vi "Sr530 ReadCh.vi"(0 "VISA Rsrc":refnum<visa-resource-name>="SR530", 1 "Autoscale":bool=TRUE, 5 "Channel":T1 items=["Channel 1", "X Output", "Channel 2", "Y Output", "X1", "X2", "X3", "X4", "X5", "X6", "Ch1 and Ch2", "X and Y", "X,Y,Ch1,Ch2"], 7 "Délais":u32, 9 "Check Status":bool, 11 "error in (no error)":errorcluster, 12 "Ask Correction":bool) -> (2 "Outputs":dbl[](array[numeric]), 3 "Warning":bool, 4 "Ressource VISA Out":refnum<visa-resource-name>="GPIB0::8::INSTR", 6 "Output":dbl format="%.4e", 8 "Output 2":dbl format="%.4e", 10 "Status Byte":bool[](array[boolean]), 14 "Ask Correction Out":bool, 15 "error out":errorcluster)   [LabVIEW 2019]
uses:
  <userlib>/SR530/Inputs.ctl
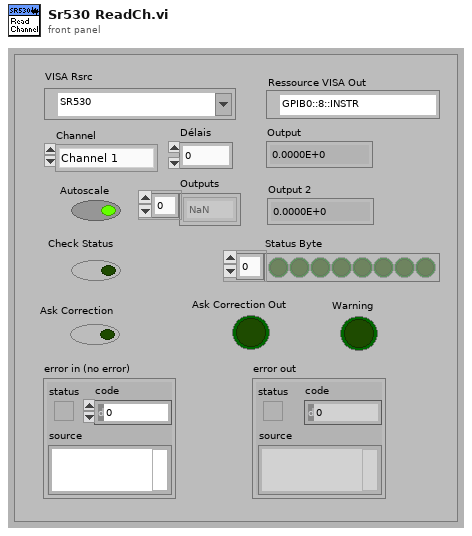
[diagram p1: front panel]
types:
  T1 = typedef "Inputs.ctl" = u16
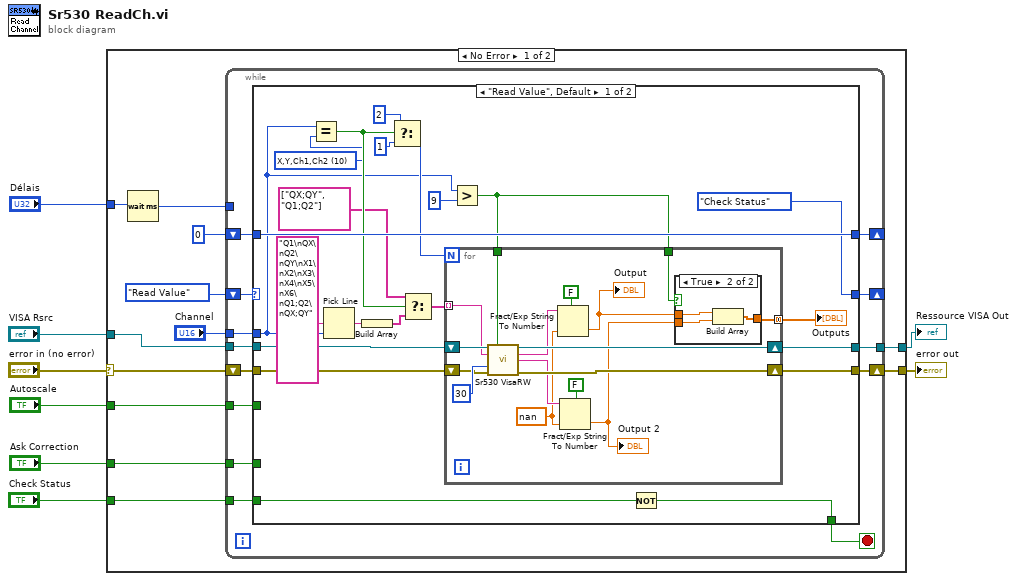
[diagram p0: block diagram]
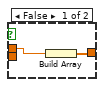
[diagram p2: hidden frame]
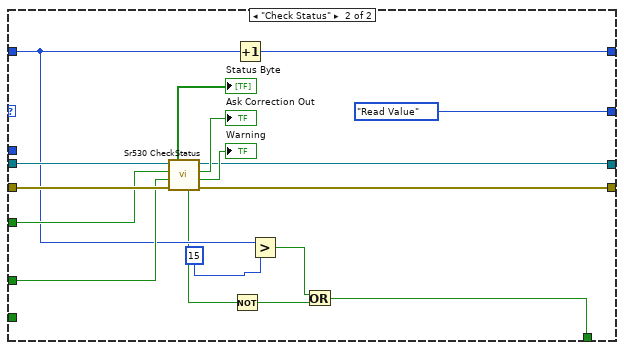
[diagram p3: hidden frame]
diagram:
  n1 = case shown="No Error" "error in (no error)" {
    selector: "error in (no error)" -> [w13 w95]
    tunnel: [w19 w95] -> w7
    tunnel: "Autoscale" -> [w18 _]
    tunnel: "Check Status" -> [w15 _]
    tunnel: "VISA Rsrc" -> [w14 w94]
    tunnel: "Ask Correction" -> [w12 _]
    tunnel: [w11 w94] -> w2
    tunnel: "Délais" -> [w10 _]
    frame No Error {
      n2 = Wait (ms)(milliseconds to wait=w10) -> (millisecond timer value=w9:u32)
      n3 = while {
        shift-right: [w29] -> _
        shift-left: enum16{"Read Value", "Check Status"}."Read Value" -> [w33]
        shift-right: [w31] -> w19
        shift-left: w13 -> [w32]
        tunnel: w18 -> [w28]
        tunnel: "Channel" -> [w27]
        shift-right: [w25] -> _
        shift-left: 0 ("timeout ms (488.2 global)") -> [w26]
        tunnel: w15 -> [w24]
        tunnel: w14 -> [w23]
        tunnel: w12 -> [w22]
        tunnel: [w21] -> w11
        tunnel: w9 -> [_]
        stop <- w30 stop-if-true
        n4 = case shown="\"Read Value\", Default" w33 {
          tunnel: w32 -> [w48 w93]
          tunnel: [w50 w91] -> w31
          tunnel: [w52 w81] -> w30
          tunnel: [enum16{"Read Value", "Check Status"}."Check Status" enum16{"Read Value", "Check Status"}."Read Value"] -> w29
          tunnel: w28 -> [_ w89]
          tunnel: w27 -> [w37 _]
          tunnel: w26 -> [w55 w83]
          tunnel: [w55 w84] -> w25
          tunnel: w24 -> [w53 _]
          tunnel: w23 -> [w47 w92]
          tunnel: w22 -> [_ w86]
          tunnel: [w51 w79] -> w21
          frame "Read Value", Default {
            w34 = T1 10 items=["Channel 1", "X Output", "Channel 2", "Y Output", "X1", "X2", "X3", "X4", "Ch1 and Ch2", "X and Y", "X,Y,Ch1,Ch2"] ("Channel")
            n5 = Equal?(x=w37, y=w34) -> (x = y?=w43:bool)
            n6 = Pick Line(multi-line string="Q1\nQX\nQ2\nQY\nX1\nX2\nX3\nX4\nX5\nX6\nQ1;Q2\nQX;QY" ("data"), line index=w37) -> (output string=w40:string)  [unwired: 1 in]
            n7 = Build Array(w40) -> (w39:string[])
            n8 = Select(t=2, s=w43, f=1) -> (s? t:f=w44:i32)
            n9 = Select(t=string[] ["QX;QY", "Q1;Q2"] ("tableau ajouté"), s=w43, f=w39) -> (s? t:f=w41:string[])
            n10 = Greater?(x=w37, y=u16 9) -> (0:w35:bool)
            n11 = for {
              N: w44 -> [_]
              tunnel: [w61] -> w49 mode=concatenating
              shift-right: [w68] -> w50
              shift-left: w48 -> [w60]
              shift-right: [w70] -> w51
              shift-left: w47 -> [w59]
              tunnel: w41 -> [w58] mode=indexing
              tunnel: w35 -> [w57]
              tunnel: w35 -> [w56]
              w64 = nan ("valeur par défaut (0 DBL)")
              n12 = call <userlib>:"Sr530 VisaRW.vi"("VISA Rsrc"=w59, "2Lecture?"=w56, "ChaineCom"=w58, "Nbcaract"=u32 30, "error in (no error)"=w60) -> ("VISA Rsrc Out"=w70:refnum<visa-resource-name>, "ChaineRep"=w69:string, "ChaineRep2"=w65:string, "error out"=w68:errorcluster)  [unwired: 5 in, 2 out]
              n13 = Fract/Exp String To Number(use system decimal point (T)=FALSE, string=w69, default (0 dbl)=w64) -> (number=w63:dbl)  [unwired: 1 in, 1 out]
              "Output" <- w63
              n14 = Fract/Exp String To Number(use system decimal point (T)=FALSE, string=w65, default (0 dbl)=w64) -> (number=w62:dbl)  [unwired: 1 in, 1 out]
              "Output 2" <- w62
              n15 = case shown="True" w57 {
                tunnel: w63 -> [w73 w76]
                tunnel: w62 -> [_ w75]
                tunnel: [w72 w74] -> w61
                frame False {
                  n16 = Build Array(w73) -> (w72:dbl[])
                }
                frame True {
                  n17 = Build Array(w76, w75) -> (w74:dbl[])
                }
              }
            }
            "Outputs" <- w49
            n18 = Not(x=w53) -> (.not. x?=w52:bool)
          }
          frame "Check Status" {
            n19 = call <userlib>:"Sr530 CheckStatus.vi"("error in (no error)"=w93, "Ask Correction"=w86, "Autoscale"=w89, "Ressource VISA In"=w92) -> ("error out"=w91:errorcluster, "Warning"=→"Warning":bool, "Ask Correction Out"=→"Ask Correction Out":bool, "Ressource VISA Out"=w79:refnum<visa-resource-name>, "Reprise"=w78:bool, "Status Byte"=→"Status Byte":bool[])
            n20 = Not(x=w78) -> (.not. x?=w77:bool)
            n21 = Increment(x=w83) -> (x+1=w84:i32)
            n22 = Greater?(x=w83, y=15) -> (0:w80:bool)
            n23 = Or(x=w80, y=w77) -> (x .or. y?=w81:bool)
          }
        }
      }
    }
    frame Error {
    }
  }
  "error out" <- w7
  "Ressource VISA Out" <- w2
